vi "Main.vi"() -> ()   [LabVIEW 2024]
uses:
  State.ctl
panel:
  in  "?":bool
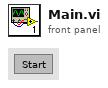
[diagram p1: front panel]
types:
  T1 = typedef "State.ctl" = enum16{"Initialize", "Standby", "Start", "Stop", "Save"}
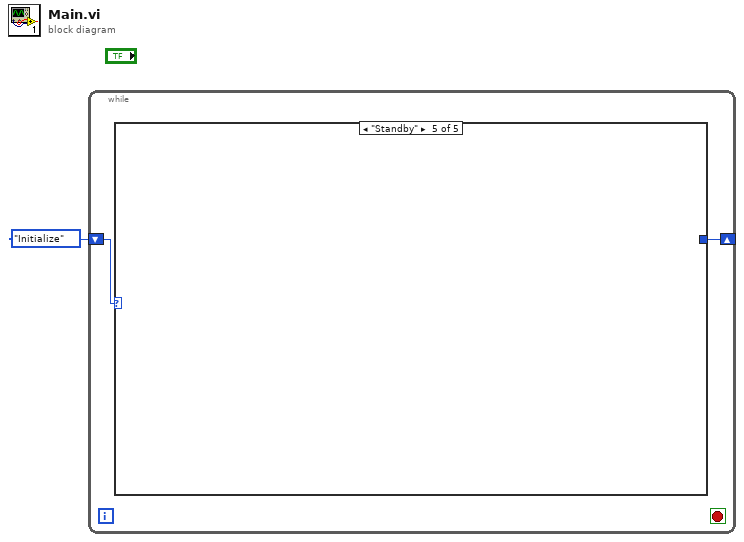
[diagram p0: block diagram]
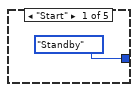
[diagram p2: hidden frame]
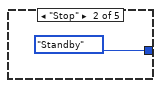
[diagram p3: hidden frame]
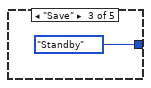
[diagram p4: hidden frame]
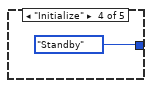
[diagram p5: hidden frame]
diagram:
  n1 = while {
    shift-right: [w3] -> _
    shift-left: State."Initialize" ("Enum") -> [w2]
    stop <- _ stop-if-true
    n2 = case shown="\"Standby\"" w2 {
      tunnel: [State."Standby" State."Standby" State."Standby" State."Standby" _] -> w3
      frame "Start" {
      }
      frame "Stop" {
      }
      frame "Save" {
      }
      frame "Initialize" {
      }
      frame "Standby" {
      }
    }
  }
